vi "Read Num1.lvclass.vi"(8 "error in (no error)":errorcluster, 11 "POffset.lvclass in":refnum<class "POffset.lvclass">) -> (0 "error out":errorcluster, 2 "Num1.lvclass":refnum<class "Num1.lvclass">, 3 "POffset.lvclass out":refnum<class "POffset.lvclass">)   [LabVIEW 2009, in "POffset.lvclass"]
uses:
  POffset.lvclass
  OffsetCommands/OffsetDef/Num1/Num1.lvclass
  POffset.lvclass/POffset.ctl
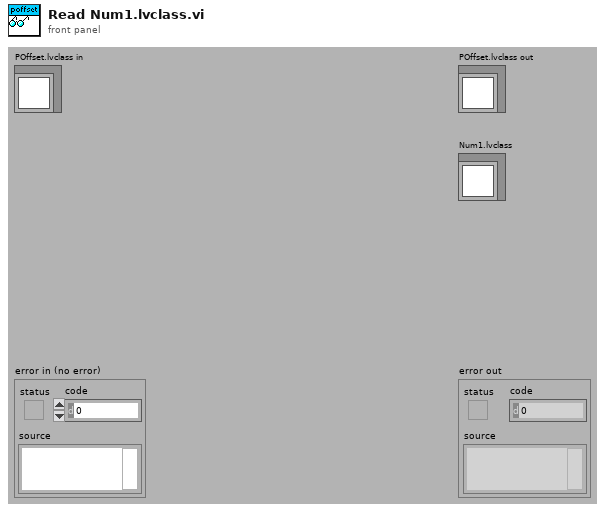
[diagram p1: front panel]
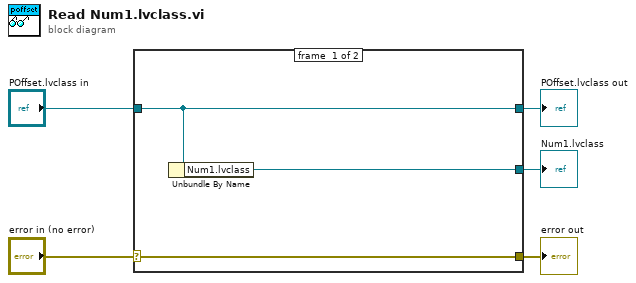
[diagram p0: block diagram]
diagram:
  n1 = case shown="No Error" "error in (no error)" {
    selector: "error in (no error)" -> [w8 w9]
    tunnel: [w8 w9] -> w4
    tunnel: [w7 w10] -> w2
    tunnel: "POffset.lvclass in" -> [w7 w10]
    tunnel: [w6 _] -> w1
    frame #0 {
      n2 = Unbundle By Name(w7) -> ("Num1.lvclass"=w6:refnum<class "Num1.lvclass">)
    }
    frame #1 {
    }
  }
  "error out" <- w4
  "POffset.lvclass out" <- w2
  "Num1.lvclass" <- w1
